vi "Initialize From File.vi"(0 "NSIS Installer in":refnum<class "NSIS Installer.lvclass">) -> (4 "NSIS Installer out":refnum<class "NSIS Installer.lvclass">)   [LabVIEW 2017, in "CL_G3_VIComponentBuilder.lvlib" / "NSIS Installer.lvclass"]
doc: "Initializes the class from the NSIS script."
uses:
  NSIS Installer.lvclass
  C:/builds/Component BuilderBT/SrcDist/Exports/Exports/Export.lvclass
  Exports/Export.lvclass/Export.ctl
  NSIS Installer.lvclass/NSIS Installer.ctl
  Accessors/Write Build Time Output Directory.vi
  Exports/Accessors/Read Export Build Specification.vi
  Exports/Accessors/Write Export Operation Errors.vi
  Compound Installer/Compound_Installer.lvclass
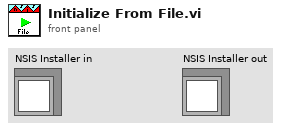
[diagram p1: front panel]
types:
  T1 = enum16{"open", "replace", "create", "open or create", "replace or create", "replace or create with confirmation"}
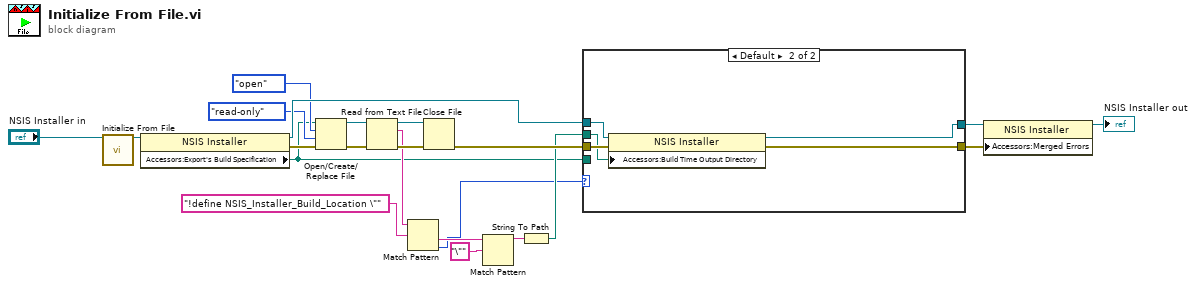
[diagram p0: block diagram]
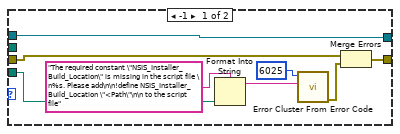
[diagram p2: hidden frame]
diagram:
  n1 = call-parent "Initialize From File.vi"("Compound_Installer in"="NSIS Installer in") -> ("Compound_Installer out"=w21:refnum<class "NSIS Installer.lvclass">)  [unwired: 14 in]
  n2 = property class="NSIS Installer"(reference=w21) -> (reference out=w20:refnum<class "NSIS Installer.lvclass">, error out=w13:errorcluster, "Accessors:Export's Build Specification"=w4:path)  [unwired: 1 in]
  n3 = Open/Create/Replace File(file path (use dialog)=w4, error in=w13, operation (0:open)=T1."open", access (0:read/write)=enum16{"read/write", "read-only", "write-only"}."read-only") -> (refnum out=w18:refnum<file>, error out=w17:errorcluster)  [unwired: 2 in, 1 out]
  n4 = Read from Text File(file (use dialog)=w18, error in=w17) -> (refnum out=w16:refnum<file>, text=w7:string, error out=w15:errorcluster)  [unwired: 2 in, 1 out]
  n5 = Match Pattern(string=w7, regular expression="!define NSIS_Installer_Build_Location \"") -> (after substring=w10:string, offset past match=w5:i32)  [unwired: 1 in, 2 out]
  n6 = Close File(refnum=w16, error in=w15) -> (error out=w12:errorcluster)  [unwired: 1 out]
  n7 = Match Pattern(string=w10, regular expression="\"") -> (before substring=w8:string)  [unwired: 1 in, 3 out]
  n8 = String To Path(string=w8) -> (path=w6:path)
  n9 = case shown="Default" w5 {
    tunnel: w20 -> [w23 w35]
    tunnel: [w23 w34] -> w1
    tunnel: w12 -> [w30 w33]
    tunnel: w6 -> [_ w32]
    tunnel: w4 -> [w25 _]
    tunnel: [w24 w31] -> w3
    frame -1 {
      n10 = Format Into String(format string="The required constant \"NSIS_Installer_Build_Location\" is missing in the script file \n%s. Please add\n\n!define NSIS_Installer_Build_Location \"<Path\"\n\n to the script file", w25) -> (resulting string=w29:string)  [unwired: 2 in, 1 out]
      n11 = call <vilib>:"Error Cluster From Error Code.vi"("error message (\"\")"=w29, "error code (0)"=6025) -> ("error out"=w27:errorcluster)  [unwired: 7 in]
      n12 = Merge Errors(w30, w27) -> (w24:errorcluster)
    }
    frame Default {
      n13 = property class="NSIS Installer"(reference=w35, error in=w33, "Accessors:Build Time Output Directory"=w32) -> (reference out=w34:refnum<class "NSIS Installer.lvclass">, error out=w31:errorcluster)
    }
  }
  n14 = property class="NSIS Installer"(reference=w1, "Accessors:Merged Errors"=w3) -> (reference out=→"NSIS Installer out":refnum<class "NSIS Installer.lvclass">)  [unwired: 1 in, 1 out]
